vi "AmpImbDemo.vi"() -> ()   [LabVIEW 2009]
uses:
  <vilib>/imath/engines/lvmath2/RunTimeEngine/ErrorHandling/NIMS_Finalize Error.vi
  <vilib>/imath/engines/lvmath2/RunTimeEngine/Parser/MC_Version.vi
  <vilib>/imathl/engines/lvmath/Functions/Error Handling/Create Error.vi
  <vilib>/imath/engines/lvmath2/RunTimeEngine/BuiltInFunctions/zeros/NIMS_M=zeros(I32,I32).vi
  <vilib>/imath/engines/lvmath2/RunTimeEngine/NodeEndStatement/NIMS_NodeEndStatement_Output.vi
  <instcachedir>/0/NIMS_NodeEndStatement_Output_53EC0D466D134D7ABD903AC30B43404B.lvgen/NIMS_NodeEndStatement_Output_53EC0D466D134D7ABD903AC30B43404B_001.vi
  <instcachedir>/0/NIMS_NodeEndStatement_Output_53EC0D466D134D7ABD903AC30B43404B.lvgen/NIMS_NodeEndStatement_Output_53EC0D466D134D7ABD903AC30B43404B_000.vi
  <vilib>/imath/engines/lvmath2/RunTimeEngine/RangeToken/NIMS_Range.vi
  <instcachedir>/0/NIMS_Range_08574DECC23E450FAF0AC0BC39E6BEA7.lvgen/NIMS_Range_08574DECC23E450FAF0AC0BC39E6BEA7_001.vi
  <vilib>/imath/engines/lvmath2/RunTimeEngine/ArithmeticOperatorToken/NIMS_ArithmeticOperator_plus.vi
  <instcachedir>/0/NIMS_ArithmeticOperator_plus_48B9519178ED42D7840F01273E784BFE.lvgen/NIMS_ArithmeticOperator_plus_48B9519178ED42D7840F01273E784BFE_001.vi
  <vilib>/imath/engines/lvmath/Functions/Error Handling/MergeErrorsWrapper.vi
  <vilib>/imath/engines/lvmath/Functions/Error Handling/MC_Error Cluster From Error Code.vi
  <vilib>/imath/engines/lvmath2/RunTimeEngine/BuiltInFunctions/fft/NIMS_fft(GV).vi
  <instcachedir>/0/NIMS_fft(GV)_4C6467FC22F84E4BA42517A07EF978B0.lvgen/NIMS_fft(GV)_4C6467FC22F84E4BA42517A07EF978B0_000.vi
  <vilib>/imath/engines/lvmath2/RunTimeEngine/BuiltInFunctions/abs/NIMS_abs(signed).vi
  <instcachedir>/0/NIMS_abs(signed)_C4FCB8E6058B49B797C7C8D53CA5F6EC.lvgen/NIMS_abs(signed)_C4FCB8E6058B49B797C7C8D53CA5F6EC_000.vi
  <vilib>/imath/engines/lvmath2/RunTimeEngine/VariableToken/Read/NIMS_Get Elements - RV(_) - Check(_).vi
  <instcachedir>/0/NIMS_Get Elements - RV(_) - Check(_)_FD08F12CA9A340B3A4DC1D5FF02404A0.lvgen/NIMS_Get Elements - RV(_) - Check(_)_FD08F12CA9A340B3A4DC1D5FF02404A0_001.vi
  <instcachedir>/0/NIMS_Get Elements - RV(_) - Check(_)_FD08F12CA9A340B3A4DC1D5FF02404A0.lvgen/NIMS_Get Elements - RV(_) - Check(_)_FD08F12CA9A340B3A4DC1D5FF02404A0_002.vi
panel:
  out "Amplitude Imbalance (V)":dbl=5.000000003975524e-09
  out "Result2 (V)":dbl=5.000000003975524e-09
  out "Resultdb2 (dB)":dbl=-166.02059990637343
  out "Power2 (W)":dbl=2.5000000039755236e-17
  out "Bin2":dbl=60.0
  in  "Next":bool
  in  "NumIterations":i32=5
  out "pwrTot (W)":dbl=0.9999999900000003
  out "pwrImbal (dB)":dbl=-166.02059990637343
  out "pwrTotdB (dB)":dbl=-4.3429447179203735e-08
  out "Resultdb (dB)":dbl=-4.3429447179203735e-08
  out "Result (V)":dbl=0.9999999950000001
  out "Power (W)":dbl=0.9999999900000003
  out "Bin":dbl=6.0
  in  "M":dbl=10.0
  in  "N":dbl=64.0
  out "Waveform Graph":dbl[](graph)=[-320.27090479940256, -331.85908592287893, -314.91628089195757, -319.1240930539387, -311.79393396068, -4.3429447179203735e-08, -312.0344339556917, -319.59087795280567, -314.87526779137266, -329.48807093121434, -321.268933630688, -321.4621010043028, -323.313106755774, -322.0786464038462, -323.02759095547054, -335.61842557423813, -324.01375944724657, -331.95806373911415, -328.66292713622715, -324.966702199033, -335.55009808182865, -324.28516139307936, -326.7363747773206, -329.121364718732, -331.83964852971883, -343.32863222152287, -329.62286550419327, -321.02950255372093, -336.5320662941356, -331.99917114879554, -323.9508139502668, -323.1836098563139, -323.5230795199891, -336.47047143432235, -319.1542857370191, -310.5732268900653, -311.5719814409753, -321.38486044085084, -311.45413714426616, -310.7299288204289, -319.73206919421324, -341.41033656840597, -323.7182233577127, -319.680444422346, -323.0177791154824, -331.6300765577489, -332.79678490810744, -322.57794702467044, -329.3305923686045, -332.98355616170556, -333.7847848074625, -326.2282360918459, -326.32055679034556, -328.89083387650896, -338.8567271819883, -322.9231917792436, -327.1090749698201, -331.1927784174165, -324.03740746398387, -166.02059990637343, -323.6984584725658, -321.33360656599854, -324.5901494406012, -319.2904618206506]
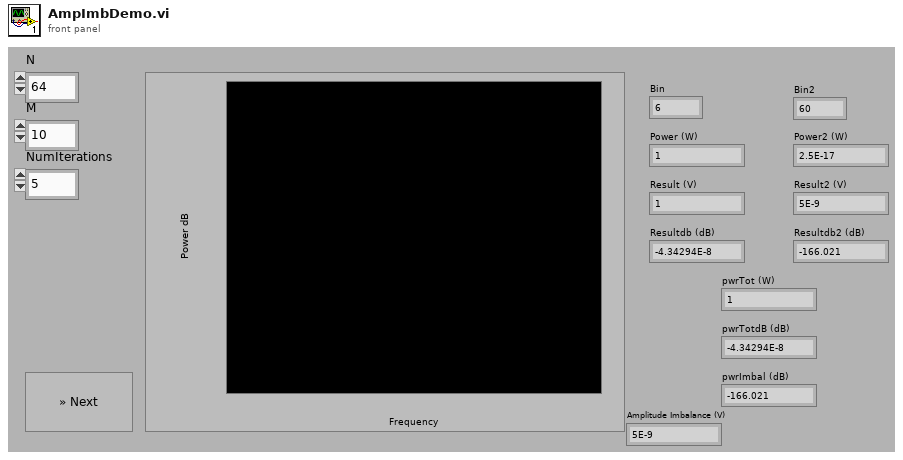
[diagram p1: front panel]
types:
  T1 = cluster{"Numeric 2":dbl, "Numeric 3":dbl, "Numeric 4":dbl}
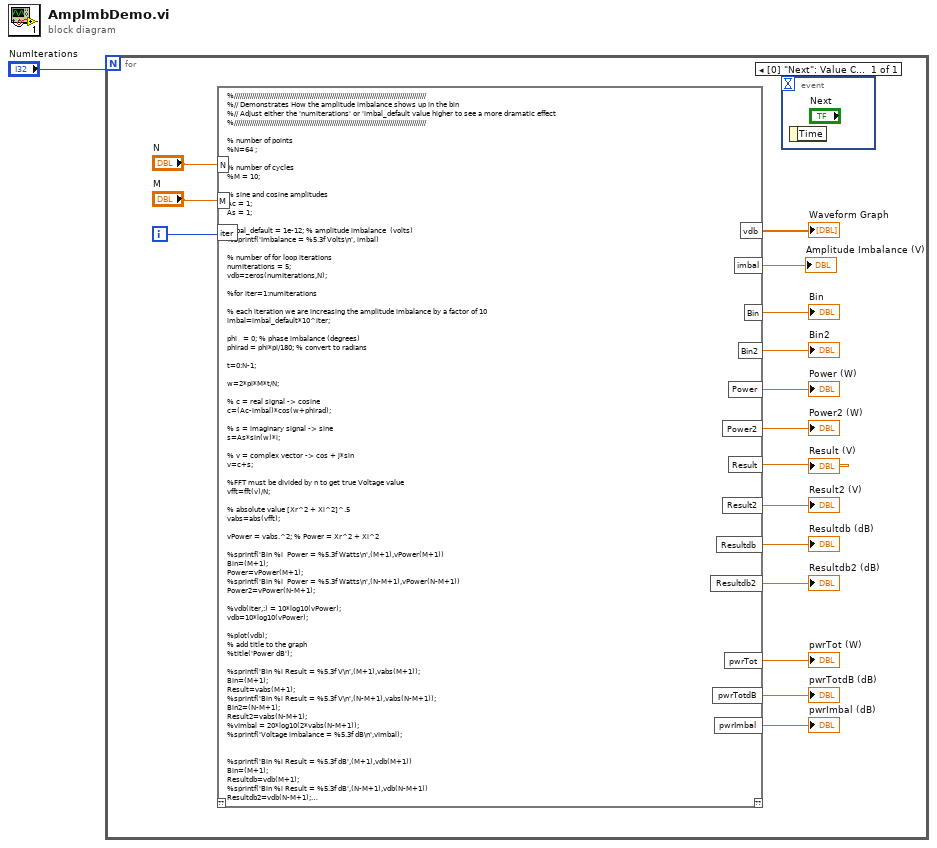
[diagram p0: block diagram]
diagram:
  n1 = for {
    N: "NumIterations" -> [_]
    i -> [w7]
    n2 = mathscript code="%////////////////////////////////////////////////////////////////////////////////////////////////\n%// Demonstrates How the amplitude imbalance shows up in the bin\n%// Adjust either the 'numIterations' or 'imbal_default value higher to see a more dramatic effect \n%////////////////////////////////////////////////////////////////////////////////////////////////\n\n% number of points\n%N=64 ;\n\n% number of cycles\n%M = 10;\n\n% sine and cosine amplitudes\nAc = 1;\nAs = 1;\n\nimbal_default = 1e-12; % amplitude imbalance  (volts)\n%sprintf('Imbalance = %5.3f Volts\\n', imbal)\n\n% number of for loop iterations\nnumIterations = 5;\nvdb=zeros(numIterations,N);\n\n%for iter=1:numIterations\n\n% each iteration we are increasing the amplitude imbalance by a factor of 10\nimbal=imbal_default*10^iter;\n\nphi   = 0; % phase imbalance (degrees)\nphirad = phi*pi/180; % convert to radians\n\nt=0:N-1;\n\nw=2*pi*M*t/N;\n\n% c = real signal -> cosine\nc=(Ac-imbal)*cos(w+phirad);\n\n% s = imaginary signal -> sine\ns=As*sin(w)*i;\n\n% v = complex vector -> cos + j*sin\nv=c+s; \n\n%FFT must be divided by n to get true Voltage value\nvfft=fft(v)/N;\n\n% absolute value [Xr^2 + Xi^2]^.5\nvabs=abs(vfft);\n\nvPower = vabs.^2; % Power = Xr^2 + Xi^2\n\n%sprintf('Bin %i  Power = %5.3f Watts\\n',(M+1),vPower(M+1))\nBin=(M+1);\nPower=vPower(M+1);\n%sprintf('Bin %i  Power = %5.3f Watts\\n',(N-M+1),vPower(N-M+1))\nPower2=vPower(N-M+1);\n\n%vdb(iter,:) = 10*log10(vPower);\nvdb=10*log10(vPower);\n\n%plot(vdb);\n% add title to the graph\n%title('Power dB');\n\n%sprintf('Bin %i Result = %5.3f V\\n',(M+1),vabs(M+1));\nBin=(M+1);\nResult=vabs(M+1);\n%sprintf('Bin %i Result = %5.3f V\\n',(N-M+1),vabs(N-M+1));\nBin2=(N-M+1);\nResult2=vabs(N-M+1);\n%vImbal = 20*log10(2*vabs(N-M+1));\n%sprintf('Voltage imbalance = %5.3f dB\\n',vImbal);\n\n\n%sprintf('Bin %i Result = %5.3f dB',(M+1),vdb(M+1))\nBin=(M+1);\nResultdb=vdb(M+1);\n%sprintf('Bin %i Result = %5.3f dB',(N-M+1),vdb(N-M+1))\nResultdb2=vdb(N-M+1);\n\npwrTot = vPower(M+1) + vPower(N-M+1);\n%sprintf('Total power = %5.3f Watts\\n',pwrTot);\n\npwrTotdB = 10*log10(pwrTot);\n%sprintf('Total power = %5.3f dB\\n',pwrTotdB)\n\npwrImbal = vdb(N-M+1);\n%sprintf('Power imbalance = %5.3f dBc\\n',pwrImbal)\n\n%end;"("N"="N", "M"="M", "iter"=w7) -> ("vdb"=→"Waveform Graph":dbl[], "Bin"=→"Bin":dbl, "Power"=→"Power (W)":dbl, "Result"=→"Result (V)":dbl, "Resultdb"=→"Resultdb (dB)":dbl, "pwrTotdB"=→"pwrTotdB (dB)":dbl, "pwrImbal"=→"pwrImbal (dB)":dbl, "pwrTot"=→"pwrTot (W)":dbl, "Bin2"=→"Bin2":dbl, "Power2"=→"Power2 (W)":dbl, "Result2"=→"Result2 (V)":dbl, "Resultdb2"=→"Resultdb2 (dB)":dbl, "imbal"=→"Amplitude Imbalance (V)":dbl)  [unwired: 1 in, 1 out]
    n3 = event shown="[0] \"Next\": Value Change" {
      selector: _ -> [_]
      dyn-events: _ -> [_]
      timeout: _ -> [_]
      event [0] "Next": Value Change {
        n4 = event-data() -> ()  [unwired: 1 in, 1 out]
      }
    }
  }
